vi "Assert Length.vi"(8 "error in":errorcluster, 10 "asserted length":u32, 11 "string in":u8[](array[numeric])) -> (0 "error out":errorcluster, 3 "Array":u8[](array[numeric]))   [LabVIEW 2020, in "NI_SFTP.lvlib" / "Low Level Connection.lvclass"]
uses:
  <vilib>/net/SFTP/Low Level Connection/Low Level Connection.lvclass
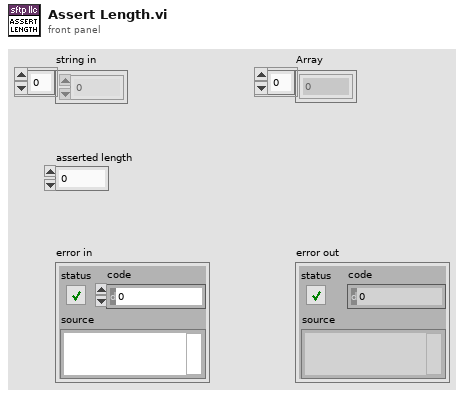
[diagram p1: front panel]
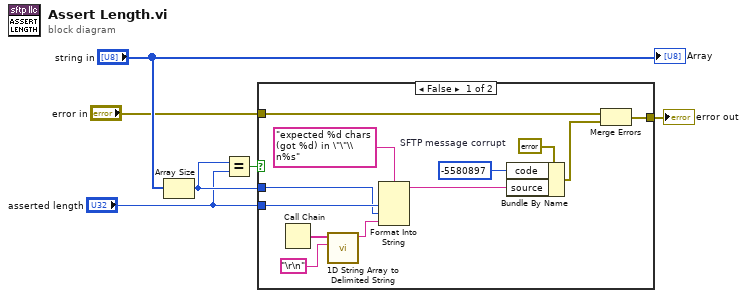
[diagram p0: block diagram]
diagram:
  n1 = Array Size(array="string in") -> (size(s)=w2:i32)
  n2 = Equal?(x=w2, y="asserted length") -> (x = y?=w5:bool)
  n3 = case shown="False" w5 {
    tunnel: [w16 w19] -> w4
    tunnel: "error in" -> [w15 w19]
    tunnel: w2 -> [w9 _]
    tunnel: "asserted length" -> [w10 _]
    frame False {
      w17 = -5580897  # SFTP message corrupt
      n4 = Call Chain() -> (call chain=w13:string[])
      n5 = call <vilib>:"1D String Array to Delimited String.vi"("delimiter"="\r\n", "string array"=w13) -> ("delimited string"=w8:string)  [unwired: 9 in]
      n6 = Format Into String(format string="expected %d chars (got %d) in \"\"\\n%s", w10, w9, w8) -> (resulting string=w7:string)  [unwired: 2 in, 1 out]
      n7 = Bundle By Name(cluster=errorcluster {"status"=TRUE, "code"=0, "source"=""} ("error in (no error)"), "code"=w17, "source"=w7) -> (w14:errorcluster)
      n8 = Merge Errors(w15, w14) -> (w16:errorcluster)
    }
    frame True {
    }
  }
  "error out" <- w4
  "Array" <- "string in"
